vi "Set Mac Address.vi"(8 "error in (no error)":errorcluster, 11 "addr":string) -> (0 "error out":errorcluster, 3 "addr out":string)   [LabVIEW 2015, in "QCA_DUT_Func.lvlib"]
doc: "DLL_QMSL_AEROFLEX void _stdcall SetMacAddress(unsigned char *addr);"
uses:
  QCA_DUT_Func.lvlib
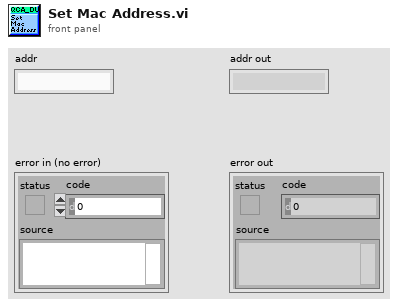
[diagram p1: front panel]
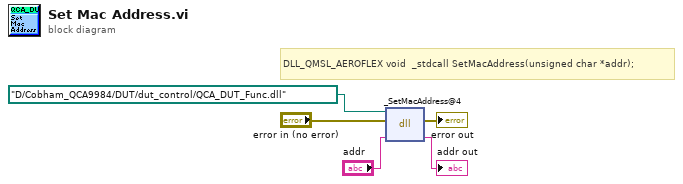
[diagram p0: block diagram]
diagram:
  # "DLL_QMSL_AEROFLEX void  _stdcall SetMacAddress(unsigned char *addr);"
  n1 = dll-call lib="D:/Cobham_QCA9984/VI/QCA_DUT_Func.dll" fn="_SetMacAddress@4"(path in=path "D:/Cobham_QCA9984/DUT/dut_control/QCA_DUT_Func.dll", error in="error in (no error)", "addr"="addr") -> (error out=→"error out":errorcluster, "addr"=→"addr out":string)  [unwired: 2 in, 1 out]
